vi "get_unit_conversions.vi"(8 "error in (no error)":errorcluster caption="错误输入（无错误）", 11 "MotorSystem输入":refnum<class "MotorSystem.lvclass">) -> (0 "error out":errorcluster caption="错误输出", 2 "unit conversions":dbl[](array[numeric]), 3 "MotorSystem输出":refnum<class "MotorSystem.lvclass">)   [LabVIEW 2016, in "MotionControl.lvlib" / "MotorSystem.lvclass"]
uses:
  <userlib>/MotionControl/MotorSystem/MotorSystem.lvclass
  <userlib>/MotionControl/MotorSystem/MotorSystem.lvclass/MotorSystem.ctl
  <userlib>/MotionControl/OneMotion/OneMotion.lvclass
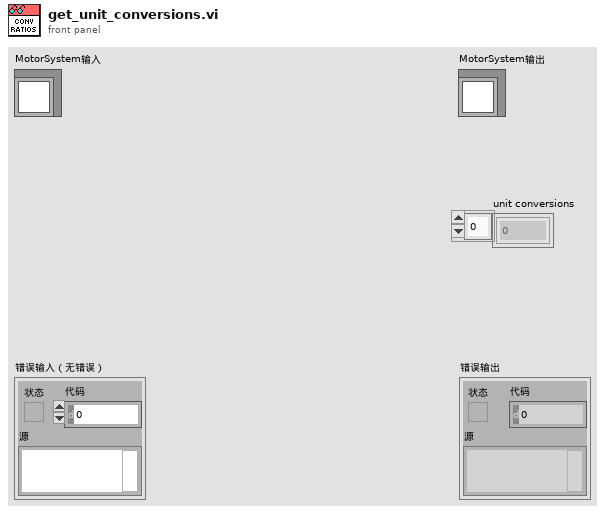
[diagram p1: front panel]
types:
  T1 = typedef "MotionControl.lvlib/MotorSystem.lvclass/MotionCluster.ctl" = cluster{"OneMotion.lvclass":refnum<class "OneMotion.lvclass">, "connected?":bool, "default enabled?":bool, "enabled?":bool}
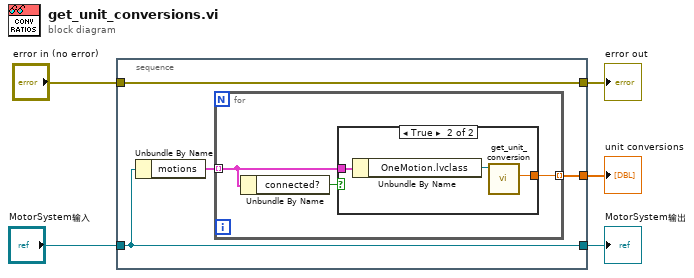
[diagram p0: block diagram]
diagram:
  n1 = stacked-sequence {
    tunnel: [w7] -> w5
    tunnel: [w9] -> w3
    tunnel: "MotorSystem输入" -> [w9]
    tunnel: "error in (no error)" -> [w7]
    tunnel: [w6] -> w1
    frame #0 {
      n2 = Unbundle By Name(w9) -> ("motions"=w8:T1[])
      n3 = for {
        tunnel: w8 -> [w11] mode=indexing
        tunnel: [w12] -> w6 mode=indexing
        n4 = Unbundle By Name(w11) -> ("connected?"=w10:bool)
        n5 = case shown="True" w10 {
          tunnel: w11 -> [_ w15]
          tunnel: [_ w13] -> w12
          frame False {
          }
          frame True {
            n6 = Unbundle By Name(w15) -> ("OneMotion.lvclass"=w14:refnum<class "OneMotion.lvclass">)
            n7 = call-dynamic "get_unit_conversion.vi"("OneMotion输入"=w14) -> ("unit conversion"=w13:dbl)  [unwired: 8 in, 2 out]
          }
        }
      }
    }
  }
  "error out" <- w5
  "MotorSystem输出" <- w3
  "unit conversions" <- w1
